vi "Get Version (uSMC).vi"(8 "error in (no error)":errorcluster, 9 "Index":i32, 11 "Visa array in":refnum<visa-resource-name>[](array[refnum])) -> (0 "error out":errorcluster, 1 "Firmware Version":string, 3 "Visa array out":refnum<visa-resource-name>[](array[refnum]))   [LabVIEW 2010, in "SignalWriterMH110203USBStepperMotor.lvclass"]
uses:
  SignalWriterMH110203USBStepperMotor.lvclass
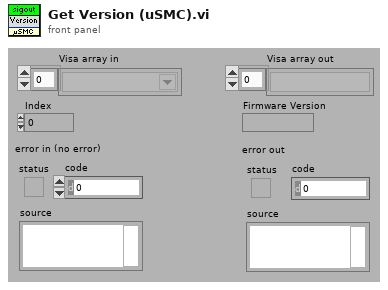
[diagram p1: front panel]
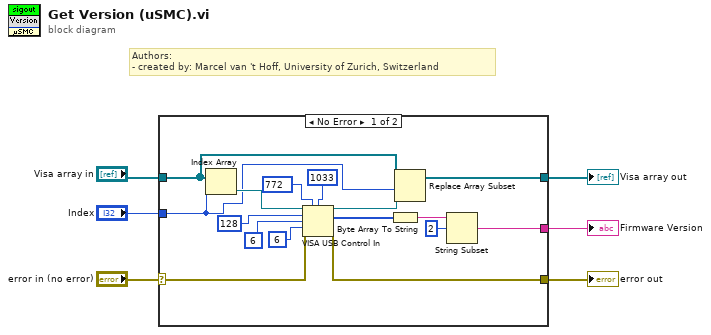
[diagram p0: block diagram]
diagram:
  # "Authors: \n- created by: Marcel van 't Hoff, University of Zurich, Switzerland"
  n1 = case shown="No Error" "error in (no error)" {
    selector: "error in (no error)" -> [w7 w23]
    tunnel: [w22 w23] -> w6
    tunnel: "Visa array in" -> [w15 w24]
    tunnel: "Index" -> [w13 _]
    tunnel: [w12 w24] -> w3
    tunnel: [w9 _] -> w2
    frame No Error {
      n2 = Index Array(array=w15, index=w13) -> (element=w16:refnum<visa-resource-name>)
      n3 = VISA USB Control In(0:w16, 1:u16 772 ("request type"), 2:u16 1033 ("request type"), 5:i16 128 ("request type"), 7:i16 6 ("request"), 9:u16 6 ("length (0)"), 11:w7) -> (4:w14:refnum<visa-resource-name>, 6:w18:u8[], 15:w22:errorcluster)
      n4 = Byte Array To String(unsigned byte array=w18) -> (string=w17:string)
      n5 = Replace Array Subset(array=w15, new element=w14, index=w13) -> (w12:refnum<visa-resource-name>[])
      n6 = String Subset(string=w17, offset (0)=2) -> (substring=w9:string)  [unwired: 1 in]
    }
    frame Error {
    }
  }
  "error out" <- w6
  "Firmware Version" <- w2
  "Visa array out" <- w3
